vi "CTRE_Phoenix_CANdle_RGBFadeAnimation.vi"(0 "CTRE_CANdle_DeviceRef":T1, 5 "Speed":dbl=1.0 min=0.0 max=1.0 step=0.0001, 7 "Num LED":i32=-1, 9 "Brightness":dbl=1.0 min=0.0 max=1.0 step=0.0001, 11 "error in":errorcluster) -> (4 "CTRE_CANdle_DeviceRef":T1, 15 "error out":errorcluster)   [LabVIEW 2020]
doc: "Animation that fades all the LEDs of a strip simultaneously between Red, Green, and Blue\n\n<b>Speed</b> adjust the speed [0,1] at which the animation runs. Valid values range from 0 to 1 where 1 is the fastest animation speed.\n\n<b>Num LEDs</b> defines the total number of LEDs to use for the animation.\n\n<b>Brightness</b> defintes how bright the animation will be [0,1]"
uses:
  <vilib>/Rock Robotics/WPI/ThirdParty/Phoenix-LabVIEW/CANdle/Controls/CTRE_Phoenix_CANdle_DeviceRef.ctl
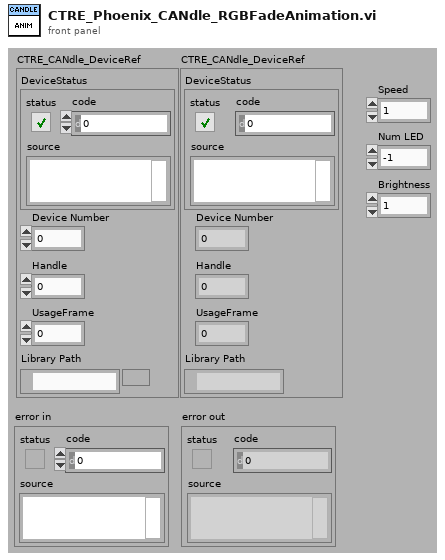
[diagram p1: front panel]
types:
  T1 = typedef "CTRE_Phoenix_CANdle_DeviceRef.ctl" = cluster{"DeviceStatus":errorcluster, "Device Number":u8, "Handle":u64, "UsageFrame":u32, "Library Path":path}
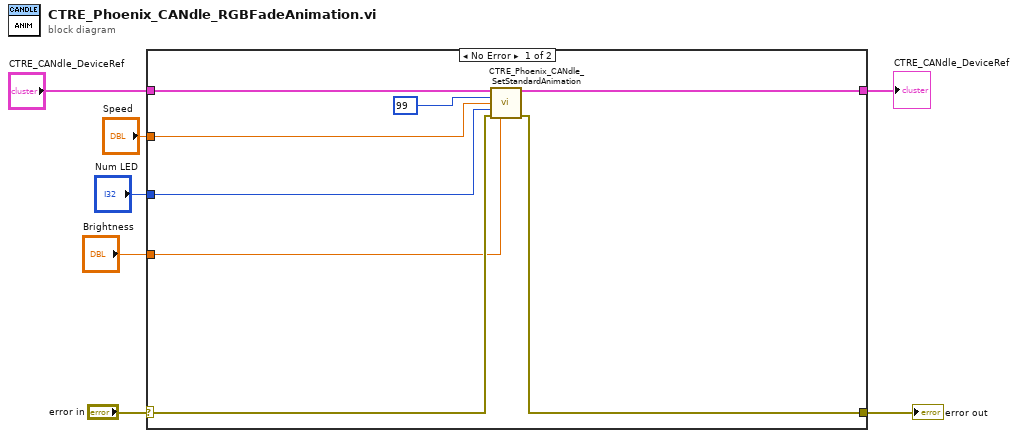
[diagram p0: block diagram]
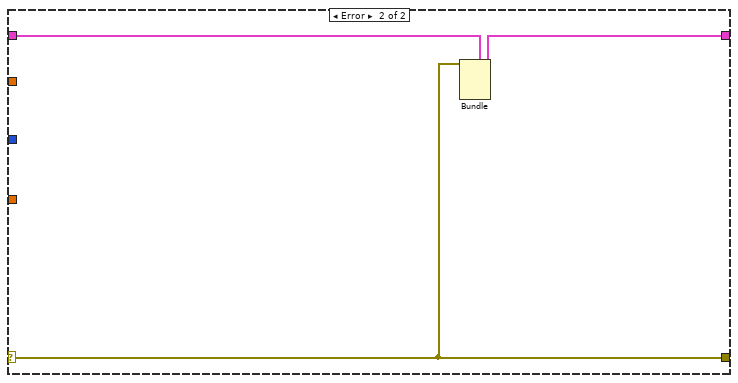
[diagram p2: hidden frame]
diagram:
  n1 = case shown="No Error" "error in" {
    selector: "error in" -> [w11 w17]
    tunnel: "CTRE_CANdle_DeviceRef" -> [w15 w18]
    tunnel: [w10 w17] -> w7
    tunnel: [w9 w16] -> w4
    tunnel: "Speed" -> [w13 _]
    tunnel: "Num LED" -> [w12 _]
    tunnel: "Brightness" -> [w8 _]
    frame No Error {
      n2 = call <vilib>:"CTRE_Phoenix_CANdle_SetStandardAnimation.vi"("CTRE_CANdle_DeviceRef"=w15, "idx"=99, "speed"=w13, "numLED"=w12, "error in"=w11, "brightness"=w8) -> ("CTRE_CANdle_DeviceRef"=w9:T1, "error out"=w10:errorcluster)  [unwired: 8 in]
    }
    frame Error {
      n3 = Bundle(cluster=w18, "DeviceStatus"=w17) -> (w16:T1)  [unwired: 4 in]
    }
  }
  "error out" <- w7
  "CTRE_CANdle_DeviceRef" <- w4
